vi "EAGLE Scanner Example.vi"   [LabVIEW 2015]
uses:
  IP Dev Area/IP results.ctl
  <vilib>/FPGAPlugInAG/cRIO-9030/niLvFpga_Open_cRIO-9030.vi
  <vilib>/rvi/interface/common/dynamic/niFpgaDynamicAddResources.vi
  <vilib>/FPGAPlugInAG/Dynamic/niLvFpga_Run_Dynamic.vi
  <vilib>/Utility/error.llb/Error Cluster From Error Code.vi
  <vilib>/rvi/errors/niLvFpgaAdjustHostInterfaceError.vi
  <vilib>/rvi/interface/nirviOpenFPGA/nirviOpenFPGA.xnode
  FPGA Bitfiles/BELKINEAGLEGUI_FPGATarget_EagleFPGAScanner_lK+EHUuZRCQ.lvbitx
  <vilib>/rvi/interface/nirviMethod/nirviMethod.xnode
  <vilib>/rvi/interface/nirviReadWriteControl/nirviReadWriteControl.xnode
  NiFpgaLv.dll
  <vilib>/rvi/interface/Simulation/niFpgaSimulationCallBeginRW.vi
types:
  T1 = typedef "IP results.ctl" = cluster{"X":u16, "Y":u16, "A":u16, "B":u16, "Grade":u16, "Frame#":u16}
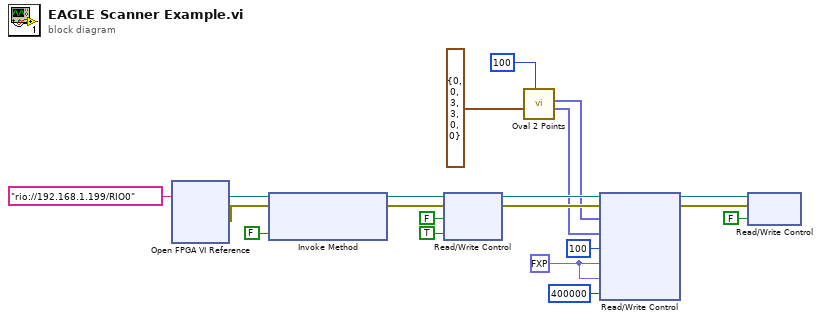
[diagram p0: block diagram]
diagram:
  w6 = fxp<+/-,20,5> 0.0 ("X OFFS")
  n1 = xnode "Open FPGA VI Reference"("resource name"=tag "rio://192.168.1.199/RIO0") -> ("FPGA VI Reference Out"=w20:refnum<k20>, "error out"=w18:errorcluster)  [unwired: 1 in]
  n2 = xnode "Invoke Method"("FPGA VI Reference In"=w20, "error in"=w18, "Wait Until Done (F)"=FALSE) -> ("FPGA VI Reference Out"=w17:refnum<k20>, "error out"=w16:errorcluster)
  n3 = xnode "Read/Write Control"("FPGA VI Reference In"=w17, "error in"=w16, "Manual"=FALSE, "Reset"=TRUE) -> ("FPGA VI Reference Out"=w13:refnum<k20>, "error out"=w12:errorcluster)
  n4 = call "Oval 2 Points .vi"("NoOfPoints"=u16 100, "IP Results"=T1 {"X"=0, "Y"=0, "A"=3, "B"=3, "Grade"=0, "Frame#"=0}) -> ("Y Points"=w7:fxp<+/-,20,5>[], "X Points"=w8:fxp<+/-,20,5>[])  [unwired: 8 in]
  n5 = xnode "Read/Write Control"("FPGA VI Reference In"=w13, "error in"=w12, "X Array"=w8, "Y Array"=w7, "NoOfPoints"=u16 100, "VX OFFS"=w6, "VY OFFS"=w6, "ScanRate"=u32 400000) -> ("FPGA VI Reference Out"=w4:refnum<k20>, "error out"=w3:errorcluster)
  n6 = xnode "Read/Write Control"("FPGA VI Reference In"=w4, "error in"=w3, "Reset"=FALSE) -> ()  [unwired: 2 out]
